vi "Stopping.vi"(9 "error in":errorcluster, 10 "Stop":bool) -> (2 "Stopping":bool, 4 "call chain":string[](array[string]))   [LabVIEW 2016]
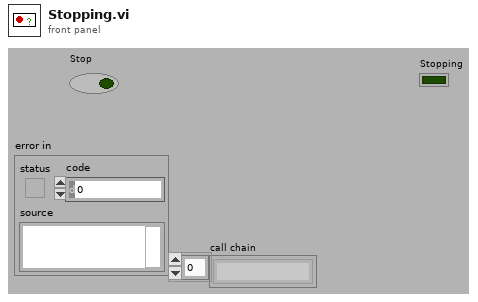
[diagram p1: front panel]
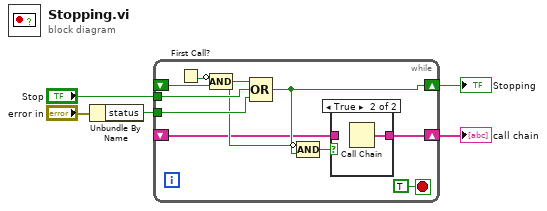
[diagram p0: block diagram]
diagram:
  n1 = Unbundle By Name("error in") -> ("status"=w3:bool)
  n2 = while {
    shift-right: [w10] -> w5
    shift-left: _ -> [w13]
    tunnel: "Stop" -> [w12]
    tunnel: w3 -> [w11]
    shift-right: [w7] -> w1
    shift-left: _ -> [w6]
    stop <- TRUE stop-if-true
    n3 = First Call?() -> (First Call?: T/F=w14:bool)
    n4 = Compound Arithmetic op=AND(invert w14, w13) -> (w9:bool)
    n5 = Compound Arithmetic op=OR(w9, w12, w11) -> (w10:bool)
    n6 = Compound Arithmetic op=AND(invert w9, w10) -> (w8:bool)
    n7 = case shown="True" w8 {
      tunnel: [w16 w17] -> w7
      tunnel: w6 -> [w16 _]
      frame False {
      }
      frame True {
        n8 = Call Chain() -> (call chain=w17:string[])
      }
    }
  }
  "Stopping" <- w5
  "call chain" <- w1
